vi "Emit If Not Empty.vi"(8 "error in (no error)":errorcluster, 10 "JSON Token Type":T1, 11 "JSON Lexer in":refnum<class "JSON Lexer.lvclass">) -> (0 "error out":errorcluster, 3 "JSON Lexer out":refnum<class "JSON Lexer.lvclass">)   [LabVIEW 2019, in "JKI JSON Serialization.lvlib" / "JSON Lexer.lvclass"]
doc: "JKI JSON 1.1.10.37\nTomi Maila - JKI\nCopyright (c) 2017, JKI"
uses:
  JSON Lexer.lvclass
  JSON Token Type.ctl
  JSON Lexer.lvclass/JSON Lexer.ctl
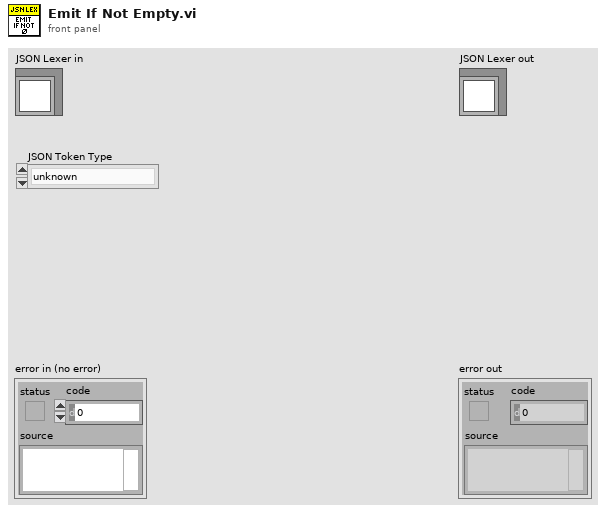
[diagram p1: front panel]
types:
  T1 = typedef "JKI JSON Serialization.lvlib/JSON Lexer.lvclass/JSON Token Type.ctl" = enum32{"unknown", "comma", "end-label", "begin-object", "end-object", "begin-array", "end-array", "quoted-string", "boolean", "exponential-number", "decimal-number", "integer-number", "special-number", "null", "symbol", "whitespace", "EOF"}
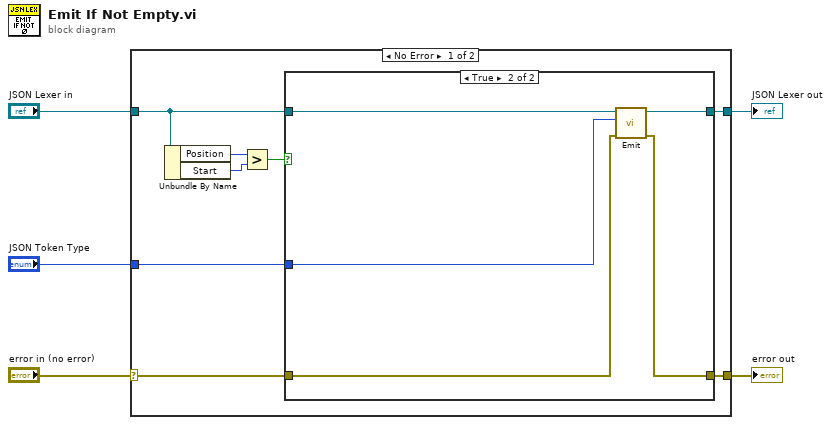
[diagram p0: block diagram]
diagram:
  n1 = case shown="No Error" "error in (no error)" {
    selector: "error in (no error)" -> [w7 w22]
    tunnel: [w6 w22] -> w4
    tunnel: [w13 w21] -> w2
    tunnel: "JSON Lexer in" -> [w12 w21]
    tunnel: "JSON Token Type" -> [w11 _]
    frame No Error {
      n2 = Unbundle By Name(w12) -> ("Position"=w10:i32, "Start"=w9:i32)
      n3 = Greater?(x=w10, y=w9) -> (0:w8:bool)
      n4 = case shown="True" w8 {
        tunnel: [w15 w20] -> w13
        tunnel: w12 -> [w15 w19]
        tunnel: w11 -> [_ w18]
        tunnel: w7 -> [w14 w17]
        tunnel: [w14 w16] -> w6
        frame False {
        }
        frame True {
          n5 = call "Emit.vi"("error in (no error)"=w17, "JSON Token Type"=w18, "JSON Lexer in"=w19) -> ("error out"=w16:errorcluster, "JSON Lexer out"=w20:refnum<class "JSON Lexer.lvclass">)  [unwired: 7 in]
        }
      }
    }
    frame Error {
    }
  }
  "error out" <- w4
  "JSON Lexer out" <- w2
